vi "Transfer.vi"(7 "Retry Delay (ms)":i32=1000, 8 "error in":errorcluster, 9 "SDO Transfer":refnum<class "SDO Transfer.lvclass">, 10 "Parameters":T2 {"Data" format="%02x"; "Multiplexer"."Sub Index" format="%02x"; "Multiplexer"."Index" format="%04x"}, 11 "SDO Manager in":refnum<class "SDO Manager.lvclass">) -> (0 "error out":errorcluster, 3 "SDO Result":T3 {"SDO abort code"."Value" items=["Toggle bit not allowed"=84082688, "SDO protocol timed out"=84148224, "Client/server command specifier not valid or unknown"=84148225, "Invalid block size (block mode only)"=84148226, "Invalid sequence number (block mode only)"=84148227, "CRC error (block mode only)"=84148228, "Out of memory"=84148229, "Attempt to read a write only object"=100728833, "Attempt to write a read only object"=100728834, "Object does not exist in the object dictionary"=100794368, "Object cannot be mapped to the PDO"=100925505, "The number and length of the objects to be mapped would exceed PDO length"=100925506, "General parameter incompatibility reason"=100925507, "General internal incompatibility in the device"=100925511, "Access failed due to an hardware error"=101056512, "Data type does not match, length of service parameter does not match"=101122064, "Data type does not match, length of service parameter too high"=101122066, "Data type does not match, length of service parameter too low"=101122067, "Sub-index does not exist"=101253137, "Invalid value for parameter (download only)"=101253168, "Value of parameter written too high (download only)"=101253169, "Value of parameter written too low (download only)"=101253170, "Maximum value is less than minimum value"=101253174, "Resource not available: SDO connection"=101318691, "General error"=134217728, "Data cannot be transferred or stored to the application"=134217760, "Data cannot be transferred or stored to the application because of local control"=134217761, "Data cannot be transferred or stored to the application because of the present device stable"=134217762, "Object dictionary dynamic generation fails or no object dictionary is present (e.g. object dictionary is generated from file and generation fails because of an file error)"=134217763, "No data available"=134217764]; "Data"."Data" format="%02x"})   [LabVIEW 2020, in "CANopen.lvlib" / "SDO Manager.lvlib" / "SDO Manager.lvclass"]
uses:
  SDO Manager.lvclass
  SDO Transfer/SDO Transfer.lvclass
  SDO Manager.lvclass/SDO Manager.ctl
  SDO Transfer/SDO Transfer.lvclass/SDO Transfer.ctl
  D:/git/CANopen-LabVIEW/source/SDO Manager/SDO Manager/SDO Transfer/SDO Transfer.lvclass
  D:/git/CANopen-LabVIEW/source/Response Matcher/IResponse/IResponse.lvclass
  Logging/Log Level.vi
  Logging/CANopen Logging.lvlib
  <vilib>/Utility/SystemLogging/NI_SystemLogging.lvlib
  SDO Transfer/SDO abort code.ctl
  Typedefs/SDO Result.ctl
  SDO Transfer/SDO Transfer Result.ctl
  Typedefs/Multiplexer.ctl
  CANopen.lvlib
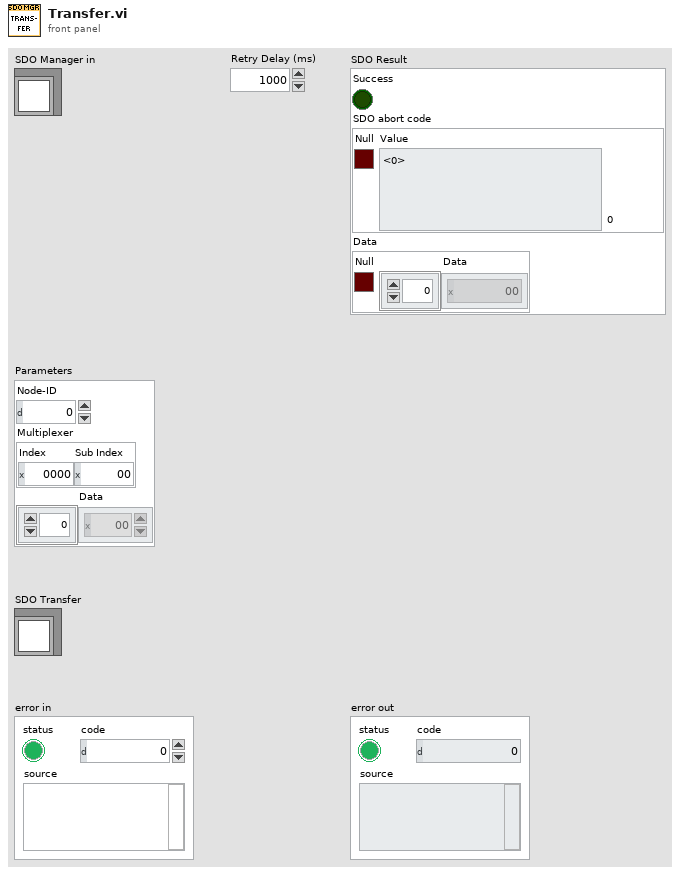
[diagram p1: front panel]
types:
  T1 = typedef "CANopen.lvlib/Multiplexer.ctl" = cluster{"Index":u16, "Sub Index":u8}
  T2 = cluster{"Node-ID":u8, "Multiplexer":T1, "Data":u8[]}
  T3 = typedef "CANopen.lvlib/SDO Manager.lvlib/SDO Transfer.lvclass/SDO Result.ctl" = cluster{"Success":bool, "SDO abort code":cluster{"Null":bool, "Value":T4}, "Data":cluster{"Null":bool, "Data":u8[]}}
  T4 = typedef "CANopen.lvlib/SDO Manager.lvlib/SDO Transfer.lvclass/SDO abort code.ctl" = u32
  T5 = typedef "CANopen.lvlib/SDO Manager.lvlib/SDO Transfer.lvclass/SDO Transfer Result.ctl" = cluster{"SDO Result":T3, "Error":errorcluster}
  T6 = enum16{"Error", "Warn", "Info", "Debug", "Trace"}
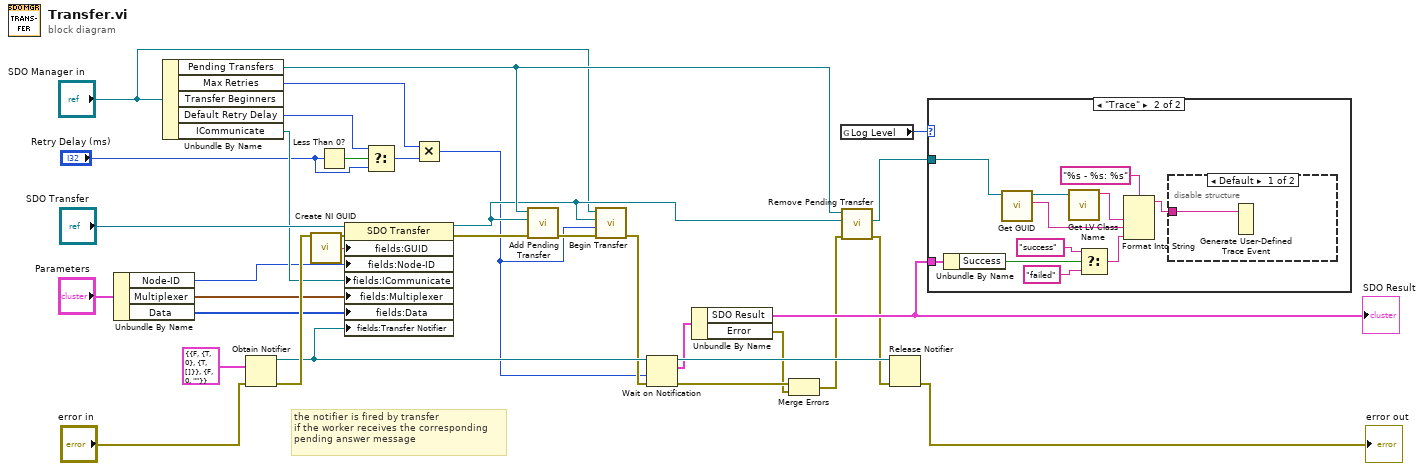
[diagram p0: block diagram]
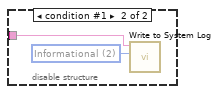
[diagram p3: hidden frame]
diagram:
  # "the notifier is fired by transfer\nif the worker receives the corresponding\npending answer message"
  n1 = Unbundle By Name("Parameters") -> ("Node-ID"=w16:u8, "Multiplexer"=w23:T1, "Data"=w1:u8[])
  n2 = Unbundle By Name("SDO Manager in") -> ("Pending Transfers"=w21:refnum<data-value>, "Max Retries"=w15:u8, "Default Retry Delay"=w29:i32, "ICommunicate"=w18:refnum<class "ICommunicate.lvclass">)  [unwired: 1 out]
  n3 = Obtain Notifier(notification data type=T5 {"SDO Result"={"Success"=FALSE, "SDO abort code"={"Null"=TRUE, "Value"=0}, "Data"={"Null"=TRUE, "Data"=[]}}, "Error"={"status"=FALSE, "code"=0, "source"=""}} ("SDO Transfer Result"), error in (no error)="error in") -> (notifier out=w30:refnum<notifier>, error out=w31:errorcluster)  [unwired: 2 in, 1 out]
  n4 = call <vilib>:"Create NI GUID.vi"() -> ("NI GUID"=w8:string)
  n5 = Less Than 0?(x="Retry Delay (ms)") -> (x < 0?=w28:bool)
  n6 = property class="SDO Transfer"(reference="SDO Transfer", error in=w31, "fields:GUID"=w8, "fields:Node-ID"=w16, "fields:ICommunicate"=w18, "fields:Multiplexer"=w23, "fields:Data"=w1, "fields:Transfer Notifier"=w30) -> (reference out=w11:refnum<class "SDO Transfer.lvclass">, error out=w32:errorcluster)
  n7 = Select(t=w29, s=w28, f="Retry Delay (ms)") -> (s? t:f=w14:i32)
  n8 = Multiply(x=w15, y=w14) -> (x*y=w9:i32)
  n9 = call "Add Pending Transfer.vi"("error in"=w32, "SDO Transfer"=w11, "Pending Transfers"=w21) -> ("error out"=w13:errorcluster)  [unwired: 8 in]
  n10 = call "Begin Transfer.vi"("error in"=w13, "Retry Delay"=w9, "SDO Transfer in"=w11, "SDO Manager"="SDO Manager in") -> ("error out"=w12:errorcluster)  [unwired: 7 in]
  n11 = Wait on Notification(notifier=w30, timeout in ms (-1)=w9, error in (no error)=w12) -> (notifier out=w33:refnum<notifier>, notification=w22:T5, error out=w19:errorcluster)  [unwired: 1 in, 1 out]
  n12 = Unbundle By Name(w22) -> ("SDO Result"=w6:T3, "Error"=w3:errorcluster)
  "SDO Result" <- w6
  n13 = Merge Errors(w19, w3) -> (w4:errorcluster)
  n14 = global read "Log Level.vi" "Log Level"() -> (w20:T6)
  n15 = call "Remove Pending Transfer.vi"("error in"=w4, "SDO Transfer"=w11, "Pending Transfers"=w21) -> ("error out"=w5:errorcluster, "Removed SDO Transfer"=w17:refnum<class "SDO Transfer.lvclass">)  [unwired: 7 in]
  n16 = Release Notifier(notifier=w33, error in (no error)=w5) -> (error out=→"error out":errorcluster)  [unwired: 1 in, 2 out]
  n17 = case shown="\"Trace\"" w20 {
    tunnel: w6 -> [_ w44]
    tunnel: w17 -> [_ w36]
    frame Default {
    }
    frame "Trace" {
      n18 = Unbundle By Name(w44) -> ("Success"=w40:bool)
      n19 = call "Get GUID.vi"("SDO Transfer in"=w36) -> ("GUID"=w34:string, "SDO Transfer out"=w35:refnum<class "SDO Transfer.lvclass">)  [unwired: 8 in, 1 out]
      n20 = call <vilib>:"Get LV Class Name.vi"("object"=w35) -> ("class name"=w42:string)  [unwired: 9 in, 1 out]
      n21 = Select(t="success", s=w40, f="failed") -> (s? t:f=w41:string)
      n22 = Format Into String(format string="%s - %s: %s" ("string"), w42, w34, w41) -> (resulting string=w37:string)  [unwired: 2 in, 1 out]
      n23 = disable-structure shown="Default" {
        disable-tunnel: w37 -> [w45 w47]
        frame condition #0 (active) {
          n24 = Generate User-Defined Trace Event(2:w45) -> ()  [unwired: 1 in]
        }
        frame condition #1 {
          w46 = 2 items=["Error", "Warning", "Informational"] ("severity")
          n25 = call <vilib>:"Write to System Log.vi"("severity"=w46, "message"=w47) -> ()  [unwired: 9 in, 1 out]
        }
      }
    }
  }
